vi "Collect_Info.vi"(5 "HART ports":refnum<visa-resource-name>[](array[refnum]), 7 "485 Ports":refnum<visa-resource-name>[](array[refnum]), 10 "MODBUS Serial Parameters":T7={"Mode"=enum."RTU", "Default Slave Address"=111, "MODBUS timeout"=1000, "Baud Rate"=38400, "Parity"=0, "Flow Control"=0} {"Flow Control" items=["None", "XON/XOFF", "RTS/CTS", "XON/XOFF & RTS/CTS", "DTR/DSR", "XON/XOFF & DTR/DSR"]; "Parity" items=["None", "Odd", "Even", "Mark", "Space"]}) -> (1 "Read Completed":bool, 2 "Information":T8, 3 "Byte order":T1(ring))   [LabVIEW 2016]
uses:
  Controls/Flow Tube Material.ctl
  Controls/mass flow unit codes.ctl
  Controls/Density Unit codes.ctl
  Controls/Temperature units.ctl
  Controls/Flow direction codes.ctl
  Controls/Information_tab_type.ctl
  OPC Server/MODBUS/MODBUS parameters type.ctl
  <vilib>/DeviceNet/VIAPI/subVIs/DnetIntfConfig.ctl
  OPC Server/Typedef/Array_of_Comm_mode_and_address_types.ctl
  OPC Server/Typedef/Comm_mode_and_address_type.ctl
  OPC Server/Typedef/Comm_mode_type_combo.ctl
  OPC Server/Protocol Class/Protocol.lvclass
  OPC Server/MASTER_OPC.ctl
  OPC Server/Typedef/event var.ctl
  OPC Server/Typedef/Comm ui action type.ctl
  OPC Server/Typedef/Comm_State_enum.ctl
  OPC Server/Typedef/state var.ctl
  OPC Server/MODBUS/MODBUS Class/MODBUS.lvclass
  C:/Users/d/Desktop/Software/Micromotion/Mark Lee/Source (1.10 US LV 2016) Branch Rabi/Blackbox/OPC Server/Protocol Class/Protocol.lvclass
  OPC Server/HART/HART Class/HART.lvclass
  OPC Server/Profibus/Profibus Class/Profibus.lvclass
  OPC Server/DeviceNET/DeviceNET Class/DeviceNET.lvclass
  OPC Server/Typedef/Protocol_enum_type.ctl
  <vilib>/DeviceNet/DeviceNetLIB.lvlib
panel:
  in  "MDOT":string="H2O"
  in  "Meter inlet static pressure (psia)":dbl
  in  "Fluid":string="H2O"
  in  "Product code*":string
  in  "Order number":string
  in  "Status *":enum32{"As found", "As left"}(radio)
  in  "Ref meter serial number*":string
  in  "Technician Name*":string
  in  "Customer Address":string
  in  "Customer Name":string
  in  "Done":bool
  out "status":bool
  in  "Protocol selection\n(appended)":T2=[{"address"=111, "Mode"=0}, {"address"=0, "Mode"=2}] {"Mode" items=["MODBUS", "HART", ""]}
  in  "Interface Name":T5(ring)
  in  "DeviceNet Interface Configuration":T6={"interface MAC ID"=0, "baud rate"=enum."500000", "poll mode"=enum."Automatic"} {"interface MAC ID" max=63 step=1}
  in  "Profibus Baud rate":i32(listbox)=6
  in  "Profibus ResourceName":refnum<visa-resource-name>="PXI5::11::INSTR"
  in  "Read":bool
  in  "Test Comments":string
  out "Test date and time":string
  out "Meter Zero":string
  in  "Meter Nominal Flow Rate (kg/min)*":string
  in  "Meter Density Repeatability":string
  in  "Meter Density Accuracy":string
  in  "Meter Zero Stability (kg/min) *":string
  in  "Meter flow repeatability":string
  in  "Meter flow accuracy (%) *":string
  out "Frequency span":string
  out "Frequency flow rate":string
  out "Flow direction":T9 items=["Forward flow only", "Reverse flow only", "Bidirectiona flow", "Absolute forward/reverse", "Negate/Forward only", "Negate/Bidirectional"]
  out "Mass flow damping":string
  out "Mass flow cutoff":string
  out "Temperature Units":T10 items=["Degrees Celsius"=32, "Degrees Fahrenheit"=33, "Degrees Rankine"=34, "Degrees Kelvin"=35, ""=0]
  out "Density units":T11 items=["Specific gravity units"=90, "Grams/cubic centimeter"=91, "Kg/cubic meter"=92, "Pounds/US gallon"=93, "Pounds/cubic foot"=94, "Grams/milliliter"=95, "Kg/liter"=96, "Pounds/cubic inch"=98, "Short tons/cubic yard"=99, "Degrees Baume (heavy)"=102, "Degrees Baume (light)"=103, "Degrees API"=104]
  out "Mass flow units":T12 items=["Grams/second"=70, "Grams/minute"=71, "Grams/hour"=72, "Kg/second"=73, "Kg/minute"=74, "Kg/hour"=75, "Kg/day"=76, "Metric tons/minute"=77, "Metric tons/hour"=78, "Metric tons/day"=79, "Pounds/second"=80, "Pounds/minute"=81, "Pounds/hour"=82, "Pounds/day"=83, "Short tons/minute"=84, "Short tons/hour"=85, "Short tons/day"=86, "Long tons/hour"=87, "Long tons/day"=88, "Special"=253]
  out "Transmitter Model":string
  in  "Sensor Model #":string
  in  "Transmitter Serial Number":string
  out "Density Temp Coeff":string
  out "FD":string
  out "K2":string
  out "K1":string
  out "D2":string
  out "D1":string
  out "FCF":string
  in  "Temp Rating":string
  in  "Pressure Rating":string
  out "Sensor Serial Number":string
  out "Flow Tube Material":T13 items=["Hastelloy C-22"=3, "Monel"=4, "Tantalum"=5, "Titanium"=6, "316L Stainless Steel"=19, "Inconel"=23, "Unknown"=252, "Special"=253]
  in  "Size":string
  # "Customer Information"
  # "*Required"
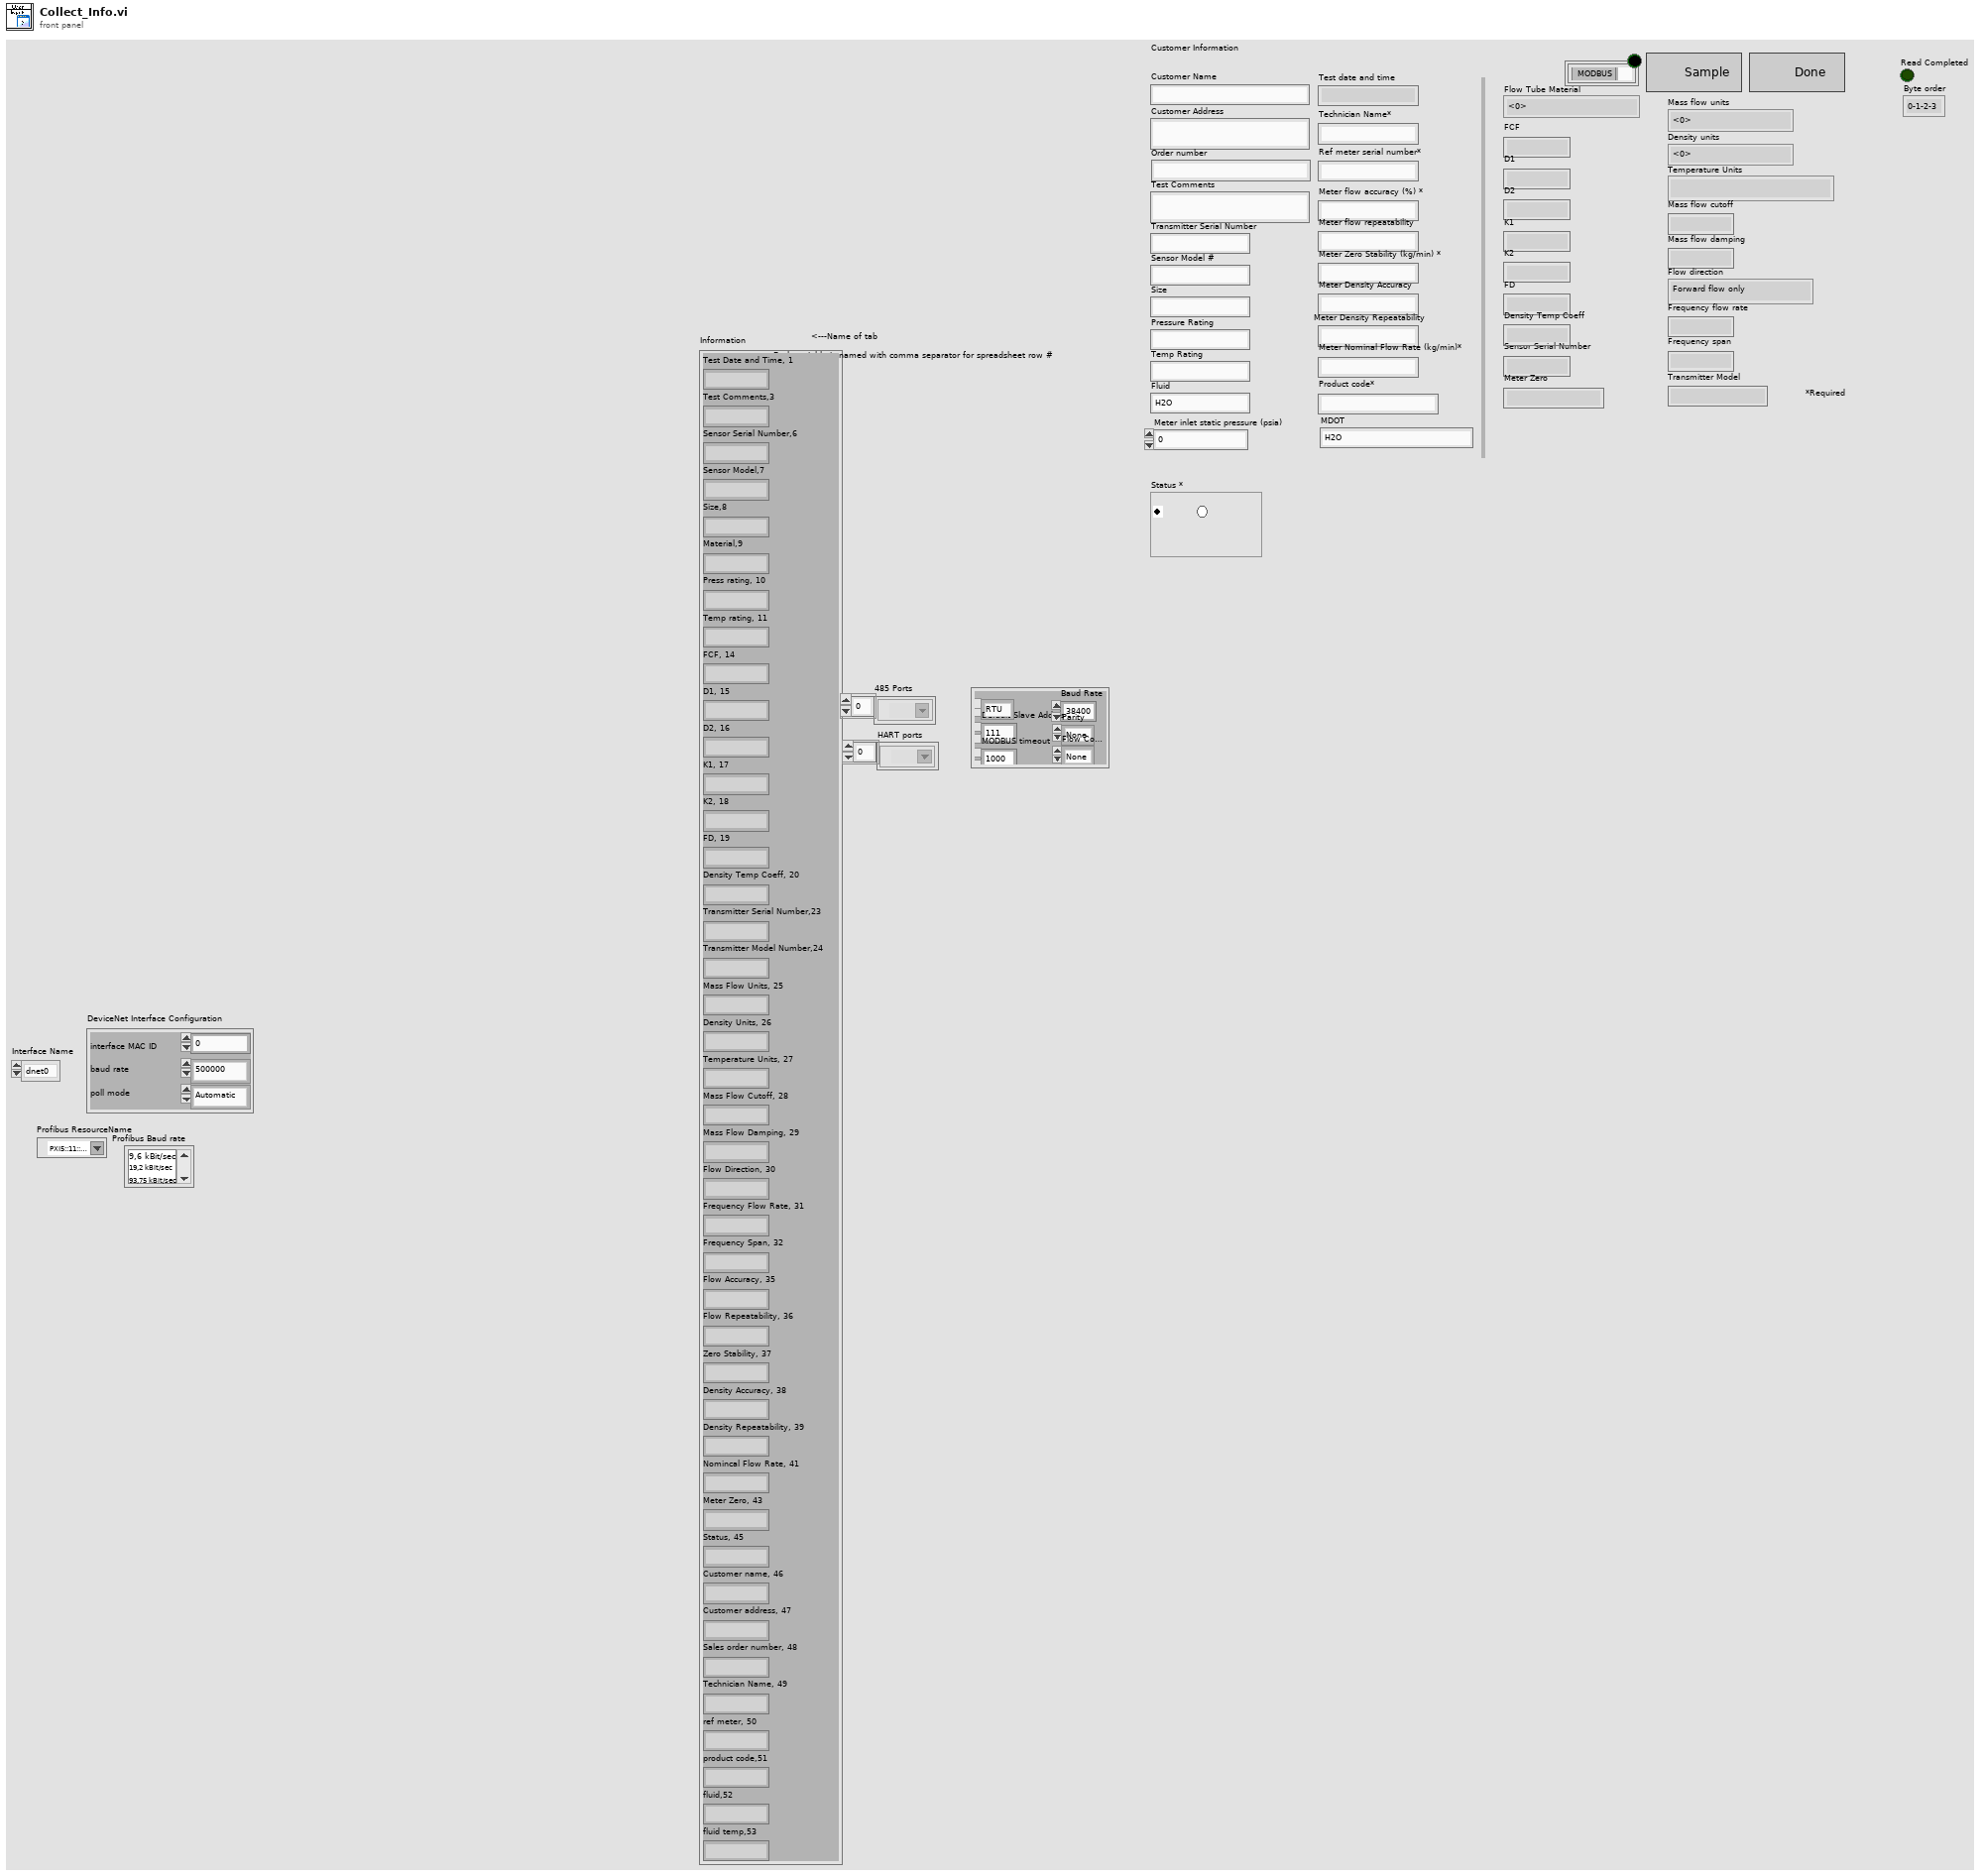
[diagram p1: front panel]
types:
  T1 = enum16{"0-1-2-3", "2-3-0-1", "1-0-3-2", "3-2-1-0"}
  T2 = typedef "Array_of_Comm_mode_and_address_types.ctl" = T3[]
  T3 = typedef "Comm_mode_and_address_type.ctl" = cluster{"address":i32, "Mode":T4}
  T4 = typedef "Comm_mode_type_combo.ctl" = u16
  T5 = enum16{"dnet0", "dnet1", "dnet2", "dnet3", "dnet4", "dnet5", "dnet6", "dnet7", "dnet8", "dnet9", "dnet10", "dnet11", "dnet12", "dnet13", "dnet14", "dnet15", "dnet16", "dnet17", "dnet18", "dnet19", "dnet20", "dnet21", "dnet22", "dnet23", "dnet24", "dnet25", "dnet26", "dnet27", "dnet28", "dnet29", "dnet30", "dnet31"}
  T6 = typedef "DeviceNetLIB.lvlib/DnetIntfConfig.ctl" = cluster{"interface MAC ID":u32, "baud rate":enum32{"125000", "250000", "500000"}, "poll mode":enum32{"Automatic", "Scanned", "Individual"}}
  T7 = typedef "MODBUS parameters type.ctl" = cluster{"Mode":enum16{"RTU", "ASCII"}, "Default Slave Address":u8, "MODBUS timeout":u32, "Baud Rate":u32, "Parity":u16, "Flow Control":u16}
  T8 = typedef "Information_tab_type.ctl" = cluster{"Test Date and Time, 1":string, "Test Comments,3":string, "Sensor Serial Number,6":string, "Sensor Model,7":string, "Size,8":string, "Material,9":string, "Press rating, 10":string, "Temp rating, 11":string, "FCF, 14":string, "D1, 15":string, "D2, 16":string, "K1, 17":string, "K2, 18":string, "FD, 19":string, "Density Temp Coeff, 20":string, "Transmitter Serial Number,23":string, "Transmitter Model Number,24":string, "Mass Flow Units, 25":string, "Density Units, 26":string, "Temperature Units, 27":string, "Mass Flow Cutoff, 28":string, "Mass Flow Damping, 29":string, "Flow Direction, 30":string, "Frequency Flow Rate, 31":string, "Frequency Span, 32":string, "Flow Accuracy, 35":string, "Flow Repeatability, 36":string, "Zero Stability, 37":string, "Density Accuracy, 38":string, "Density Repeatability, 39":string, "Nomincal Flow Rate, 41":string, "Meter Zero, 43":string, "Status, 45":string, "Customer name, 46":string, "Customer address, 47":string, "Sales order number, 48":string, "Technician Name, 49":string, "ref meter, 50":string, "product code,51":string, "fluid,52":string, "fluid temp,53":string}
  T9 = typedef "Flow direction codes.ctl" = u16
  T10 = typedef "Temperature units.ctl" = u16
  T11 = typedef "Density Unit codes.ctl" = u16
  T12 = typedef "mass flow unit codes.ctl" = u16
  T13 = typedef "Flow Tube Material.ctl" = u16
  T14 = typedef "MASTER_OPC.ctl" = cluster{"Main event var":refnum<user-event>, "VIRef":refnum<vi>, "Data path":path, "Reads":i32, "total number of UUT":i32, "FF refnum":cluster{"Handle1":u32, "Handle2":u32}, "FF device id list":string[], "MODBUS resource name":refnum<visa-resource-name>, "MODBUS Serial Parameters":cluster{"Mode":enum16{"RTU", "ASCII"}, "Default Slave Address":u8, "MODBUS timeout":u32, "Baud Rate":u32, "Parity":u16, "Flow Control":u16}, "Profibus resource name":refnum<visa-resource-name>, "Profibus Communication ref.:":u8, "HART resource name":refnum<visa-resource-name>, "HART long addresses (array)":u8[][], "Comm relay session":refnum<k15>, "Comm UI event":refnum<user-event>, "Write Interval (s)":dbl, "DMM_QUEUE":refnum<queue>, "POWER_QUEUE":refnum<queue>, "\nTHERM_QUEUE":refnum<queue>, "\nCOMM_QUEUE":refnum<queue>, "TIMING_QUEUE":refnum<queue>, "MAIN_QUEUE":refnum<queue>, "Log path":path}
  T15 = typedef "Protocol_enum_type.ctl" = enum16{"None", "MODBUS", "HART", "Fieldbus", "Profibus DP", "Profibus PA", "DeviceNET", "USB"}
  T16 = typedef "comm_variable_definition.ctl" = cluster{"General Parameter name":string, "MODBUS Register":i32, "Profibus":cluster{"Friendly name":string, "PA":cluster{"Slot":i32, "Index":i32}, "DP":cluster{"Slot":i32, "Index":i32}, "Tag":string}, "Fieldbus":cluster{"Parameter name":string, "Fieldbus Block":string, "Fieldbus Tag":string}, "data type":enum16{"float", "UINT", "UINT32", "STRING"}, "DeviceNET":cluster{"ClassId":u16, "InstanceId":u16, "AttributeId":u8}, "Cluster":T3, "Length":i32}
  T17 = cluster{"U16":u16, "U32":u32, "float":sgl, "string":string}
  T18 = typedef "CS_PB_DPV1_MSAC2_InitiateReqData.ctl" = cluster{"Communication ref.:":u8, "Send timeout:":u16, "Feat. supp. 1:":u8, "Feat. supp. 2:":u8, "Profile feat. supp. 1:":u8, "Profile feat. supp. 2:":u8, "Profile ID number:":u16, "Addional address parameter":cluster{"S-Type":bool, "S-Length:":u8, "D-Type":bool, "D-Length:":u8, "Data:":u8[]}}
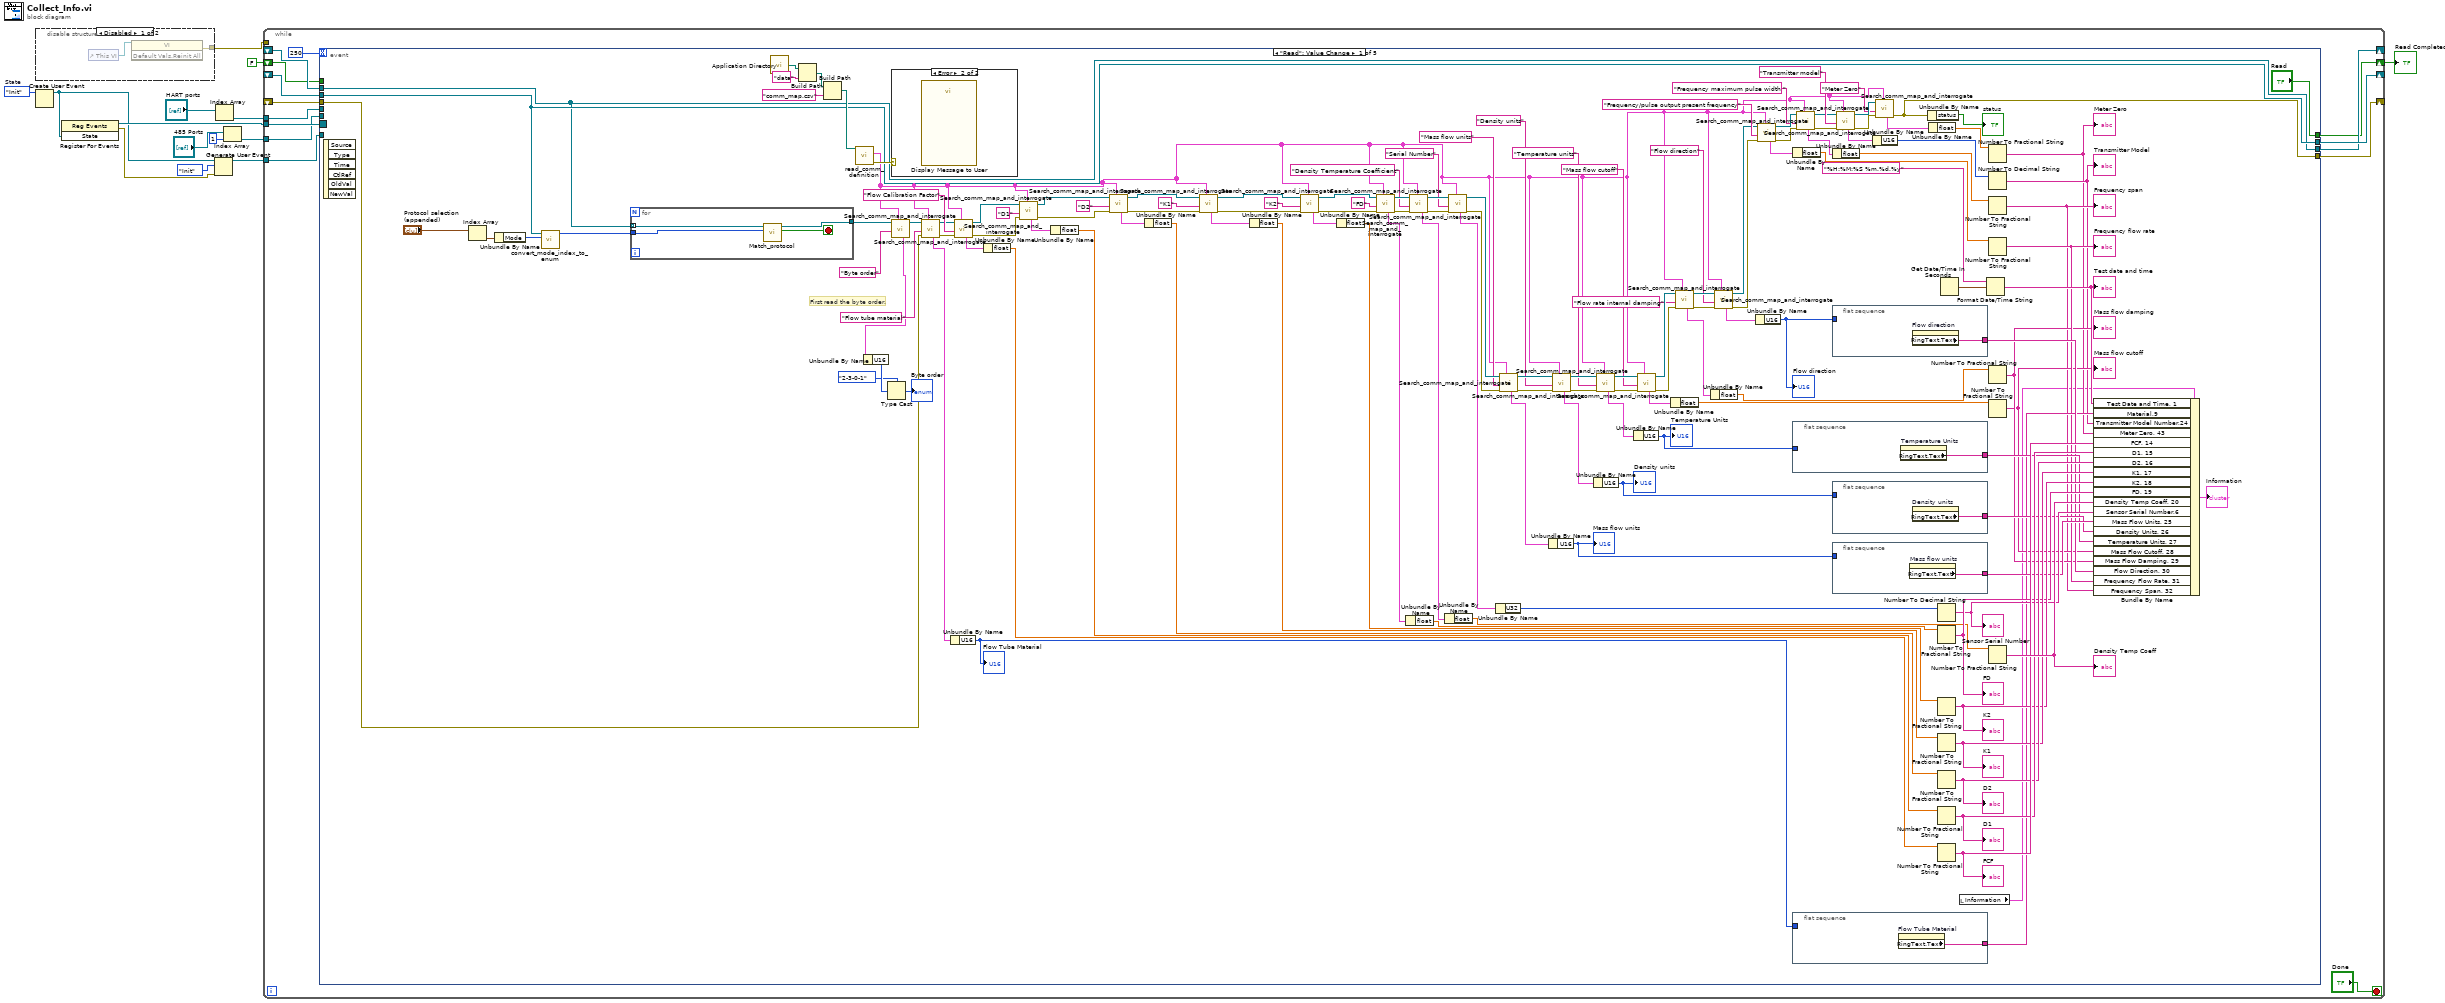
[diagram p0: block diagram]
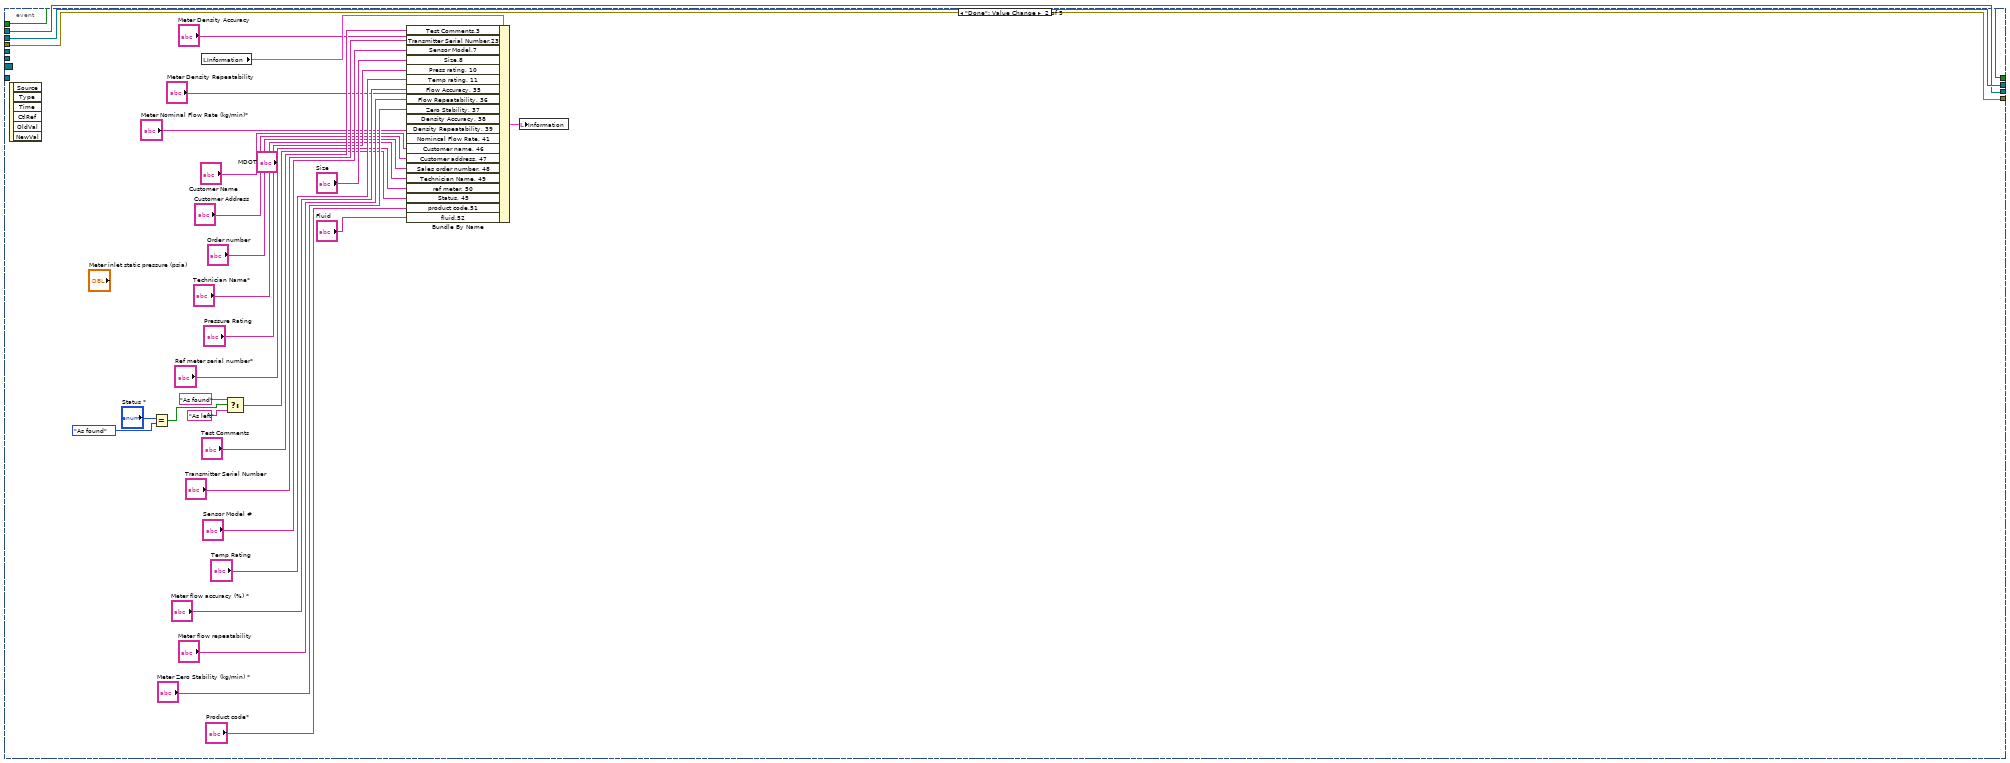
[diagram p4: hidden frame]
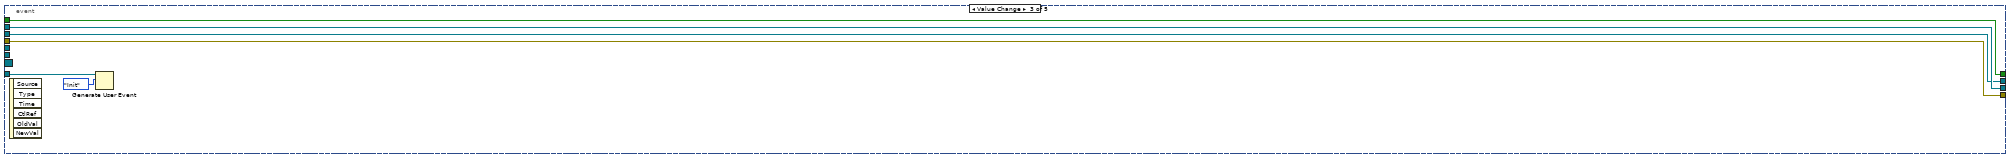
[diagram p5: hidden frame]
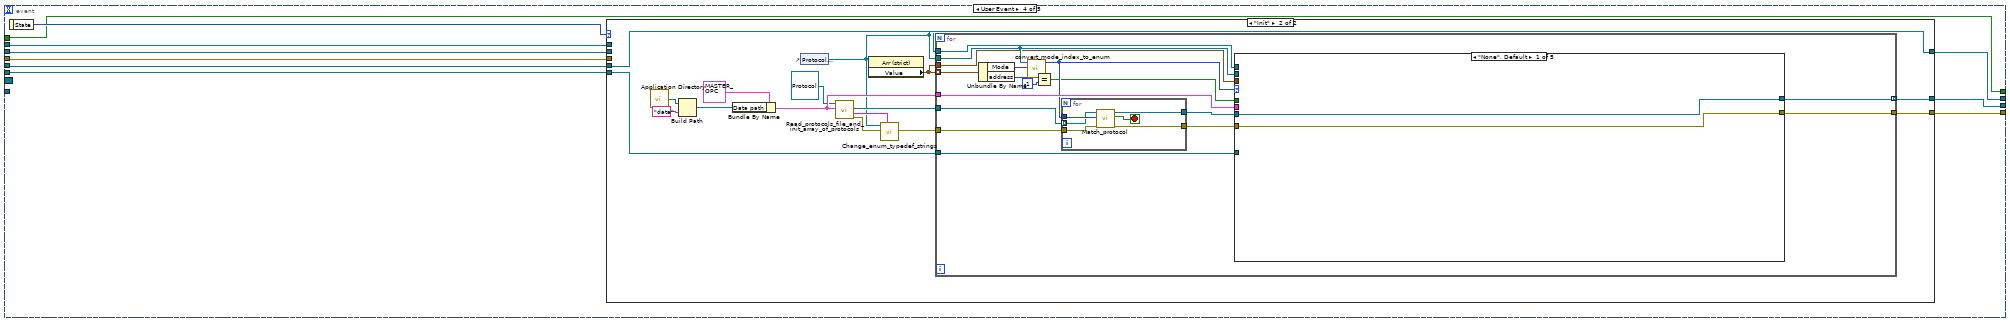
[diagram p6: hidden frame]
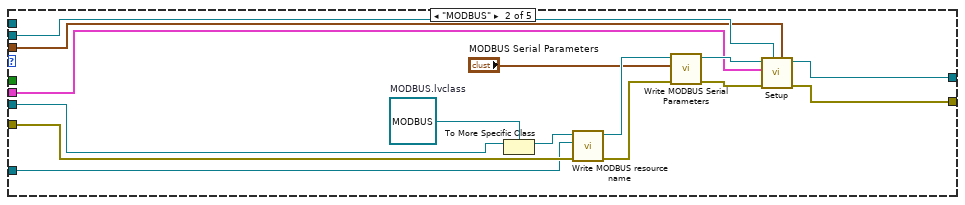
[diagram p8: hidden frame]
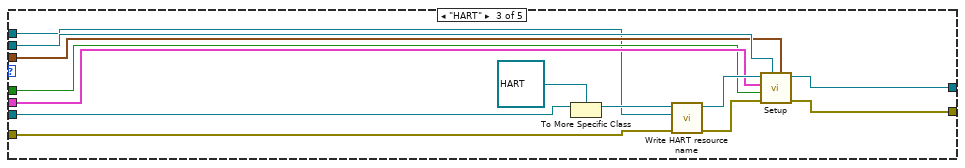
[diagram p9: hidden frame]
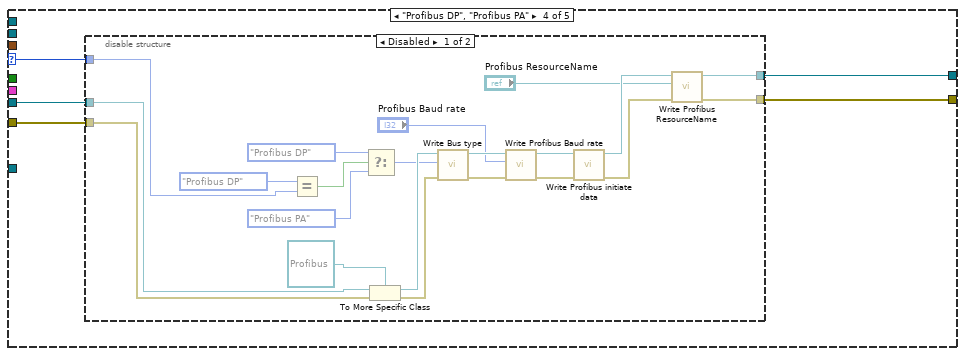
[diagram p10: hidden frame]
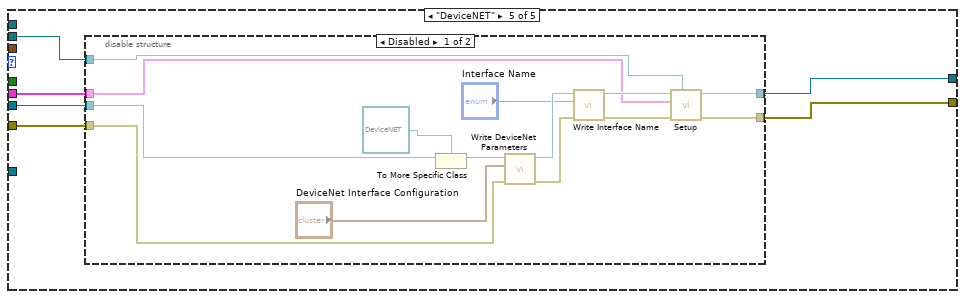
[diagram p12: hidden frame]
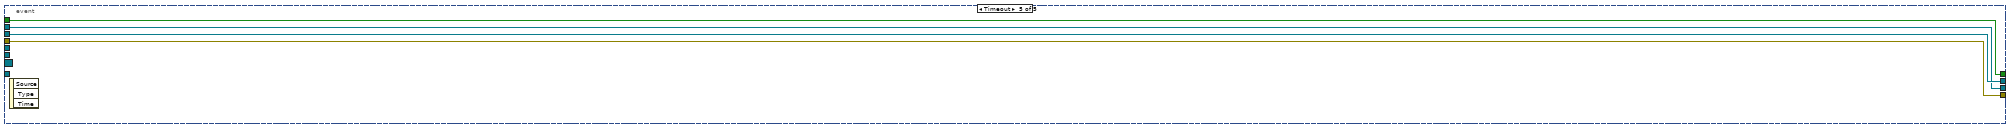
[diagram p14: hidden frame]
diagram:
  w9 = enum16{"Init", "Idle"}."Init"  # State
  n1 = disable-structure shown="Disabled" {
    disable-tunnel: [w15 _] -> w6
    frame Disabled {
      n2 = control-ref of="This VI"() -> (w16:refnum<vi>)
      n3 = invoke class="VI" method="Default Vals.Reinit All"(reference=w16) -> (error out=w15:errorcluster)  [unwired: 2 in, 2 out]
    }
    frame Enabled {
    }
  }
  n4 = Create User Event(user event datatype=w9) -> (user event=w10:refnum<user-event>)  [unwired: 1 in, 1 out]
  n5 = register-events(w10) -> (reference out=w12:refnum<event-registration>, error out=w14:errorcluster)  [unwired: 2 in]
  n6 = Generate User Event(user event=w10, event data cluster=enum16{"Init", "Idle"}."Init" ("event data"), error in=w14) -> (user event out=w11:refnum<user-event>)  [unwired: 1 in, 1 out]
  n7 = Index Array(array="HART ports") -> (element=w4:refnum<visa-resource-name>)  [unwired: 1 in]
  n8 = Index Array(array="485 Ports", index=1) -> (element=w2:refnum<visa-resource-name>)
  n9 = while {
    tunnel: w12 -> [w25]
    shift-right: [w24] -> _
    shift-left: _ -> [w28]
    shift-right: [w23] -> _
    shift-left: _ -> [w30]
    shift-right: [w22] -> _
    shift-left: _ -> [w29]
    tunnel: w11 -> [w21]
    shift-right: [w20] -> w8
    shift-left: FALSE ("Read") -> [w19]
    tunnel: w6 -> [_]
    tunnel: w4 -> [w18]
    tunnel: w2 -> [w17]
    stop <- "Done" stop-if-true
    n10 = event shown="[0] \"Read\": Value Change" {
      selector: w25 -> [_ _ _ _ _]
      dyn-events: _ -> [_ _ _ _ _]
      timeout: u32 250 ("millisecond multiple") -> [_ _ _ _ _]
      tunnel: w30 -> [w40 w210 w215 w223 w349]
      tunnel: w29 -> [w171 w209 w213 w222 w348]
      tunnel: w28 -> [w42 w211 w214 w221 w350]
      tunnel: [w42 w211 w214 w227 w350] -> w24
      tunnel: [w40 w210 w215 w226 w349] -> w23
      tunnel: [w169 w209 w213 w225 w348] -> w22
      tunnel: w21 -> [_ _ w217 _ _]
      tunnel: ["Read" w208 w212 w220 w347] -> w20
      tunnel: w19 -> [_ w208 w212 w220 w347]
      tunnel: w18 -> [_ _ _ w219 _]
      tunnel: w17 -> [_ _ _ w218 _]
      event "Read": Value Change {
        # "First read the byte order."
        n11 = event-data() -> ()  [unwired: 1 in, 6 out]
        n12 = Index Array(array="Protocol selection\n(appended)") -> (element=w44:T3)  [unwired: 1 in]
        n13 = Unbundle By Name(w44) -> ("Mode"=w43:T4)
        n14 = call "convert_mode_index_to_enum.vi"("index"=w43, "CtlRef"=w42) -> ("Protocol enum"=w41:T15)  [unwired: 6 in, 3 out]
        n15 = for {
          tunnel: w41 -> [w175]
          tunnel: w40 -> [w174] mode=indexing
          tunnel: [w172] -> w38
          stop <- w173 stop-if-true
          n16 = call-dynamic "Match_protocol.vi"("Protocol type"=w175, "Protocol in"=w174) -> ("Match"=w173:bool, "Protocol out"=w172:refnum<class "Protocol.lvclass">)  [unwired: 7 in, 1 out]
        }
        n17 = call <vilib>:"Application Directory.vi"() -> ("Application Directory"=w163:path)
        n18 = Build Path(base path=w163, name or relative path="data") -> (appended path=w159:path)
        n19 = Build Path(base path=w159, name or relative path="comm_map.csv") -> (appended path=w161:path)
        n20 = call "read_comm_definition.vi"("file path (dialog if empty)"=w161) -> ("error out"=w158:errorcluster, "Comm variable definitions"=w36:T16[])  [unwired: 8 in, 1 out]
        n21 = case shown="Error" w158 {
          frame No Error {
          }
          frame Error {
            n22 = call "Display Message to User"() -> ()  [unwired: 10 in, 2 out]
          }
        }
        n23 = call "Search_comm_map_and_interrogate.vi"("array of registers"=w36, "Register name"="Byte order", "Protocol in"=w38) -> ("Protocol out"=w37:refnum<class "Protocol.lvclass">, "output cluster"=w34:T17)  [unwired: 6 in, 1 out]
        n24 = Unbundle By Name(w34) -> ("U16"=w33:u16)
        n25 = Type Cast(type=T1."2-3-0-1" ("Byte order"), x=w33) -> (*(type *) &x=→"Byte order":T1)
        n26 = call "Search_comm_map_and_interrogate.vi"("array of registers"=w36, "error in (no error)"=w171, "Register name"="Flow tube material", "Protocol in"=w37) -> ("error out"=w78:errorcluster, "Protocol out"=w79:refnum<class "Protocol.lvclass">, "output cluster"=w77:T17)  [unwired: 5 in]
        n27 = Unbundle By Name(w77) -> ("U16"=w74:u16)
        "Flow Tube Material" <- w74
        n28 = call "Search_comm_map_and_interrogate.vi"("array of registers"=w36, "error in (no error)"=w78, "Register name"="Flow Calibration Factor", "Protocol in"=w79) -> ("error out"=w156:errorcluster, "Protocol out"=w155:refnum<class "Protocol.lvclass">, "output cluster"=w153:T17)  [unwired: 5 in]
        n29 = Unbundle By Name(w153) -> ("float"=w152:sgl)
        n30 = call "Search_comm_map_and_interrogate.vi"("array of registers"=w36, "error in (no error)"=w156, "Register name"="D1", "Protocol in"=w155) -> ("error out"=w150:errorcluster, "Protocol out"=w154:refnum<class "Protocol.lvclass">, "output cluster"=w147:T17)  [unwired: 5 in]
        n31 = Unbundle By Name(w147) -> ("float"=w148:sgl)
        n32 = call "Search_comm_map_and_interrogate.vi"("array of registers"=w36, "error in (no error)"=w150, "Register name"="D2", "Protocol in"=w154) -> ("error out"=w140:errorcluster, "Protocol out"=w141:refnum<class "Protocol.lvclass">, "output cluster"=w143:T17)  [unwired: 5 in]
        n33 = Unbundle By Name(w143) -> ("float"=w144:sgl)
        n34 = call "Search_comm_map_and_interrogate.vi"("array of registers"=w36, "error in (no error)"=w140, "Register name"="K1", "Protocol in"=w141) -> ("error out"=w134:errorcluster, "Protocol out"=w135:refnum<class "Protocol.lvclass">, "output cluster"=w138:T17)  [unwired: 5 in]
        n35 = Unbundle By Name(w138) -> ("float"=w139:sgl)
        n36 = call "Search_comm_map_and_interrogate.vi"("array of registers"=w36, "error in (no error)"=w134, "Register name"="K2", "Protocol in"=w135) -> ("error out"=w128:errorcluster, "Protocol out"=w129:refnum<class "Protocol.lvclass">, "output cluster"=w131:T17)  [unwired: 5 in]
        n37 = Unbundle By Name(w131) -> ("float"=w132:sgl)
        n38 = call "Search_comm_map_and_interrogate.vi"("array of registers"=w36, "error in (no error)"=w128, "Register name"="FD", "Protocol in"=w129) -> ("error out"=w121:errorcluster, "Protocol out"=w123:refnum<class "Protocol.lvclass">, "output cluster"=w127:T17)  [unwired: 5 in]
        n39 = Unbundle By Name(w127) -> ("float"=w125:sgl)
        n40 = call "Search_comm_map_and_interrogate.vi"("array of registers"=w36, "error in (no error)"=w121, "Register name"="Density Temperature Coefficient", "Protocol in"=w123) -> ("error out"=w118:errorcluster, "Protocol out"=w117:refnum<class "Protocol.lvclass">, "output cluster"=w119:T17)  [unwired: 5 in]
        n41 = Unbundle By Name(w119) -> ("float"=w120:sgl)
        n42 = call "Search_comm_map_and_interrogate.vi"("array of registers"=w36, "error in (no error)"=w118, "Register name"="Serial Number", "Protocol in"=w117) -> ("error out"=w112:errorcluster, "Protocol out"=w113:refnum<class "Protocol.lvclass">, "output cluster"=w115:T17)  [unwired: 5 in]
        n43 = Unbundle By Name(w115) -> ("U32"=w59:u32)
        n44 = call "Search_comm_map_and_interrogate.vi"("array of registers"=w36, "error in (no error)"=w112, "Register name"="Mass flow units", "Protocol in"=w113) -> ("error out"=w111:errorcluster, "Protocol out"=w110:refnum<class "Protocol.lvclass">, "output cluster"=w108:T17)  [unwired: 5 in]
        n45 = Unbundle By Name(w108) -> ("U16"=w104:u16)
        "Mass flow units" <- w104
        n46 = call "Search_comm_map_and_interrogate.vi"("array of registers"=w36, "error in (no error)"=w111, "Register name"="Density units", "Protocol in"=w110) -> ("error out"=w100:errorcluster, "Protocol out"=w101:refnum<class "Protocol.lvclass">, "output cluster"=w106:T17)  [unwired: 5 in]
        n47 = Unbundle By Name(w106) -> ("U16"=w102:u16)
        "Density units" <- w102
        n48 = call "Search_comm_map_and_interrogate.vi"("array of registers"=w36, "error in (no error)"=w100, "Register name"="Temperature units", "Protocol in"=w101) -> ("error out"=w95:errorcluster, "Protocol out"=w94:refnum<class "Protocol.lvclass">, "output cluster"=w98:T17)  [unwired: 5 in]
        n49 = Unbundle By Name(w98) -> ("U16"=w97:u16)
        "Temperature Units" <- w97
        n50 = call "Search_comm_map_and_interrogate.vi"("array of registers"=w36, "error in (no error)"=w95, "Register name"="Mass flow cutoff", "Protocol in"=w94) -> ("error out"=w88:errorcluster, "Protocol out"=w90:refnum<class "Protocol.lvclass">, "output cluster"=w92:T17)  [unwired: 5 in]
        n51 = Unbundle By Name(w92) -> ("float"=w91:sgl)
        n52 = call "Search_comm_map_and_interrogate.vi"("array of registers"=w36, "error in (no error)"=w88, "Register name"="Flow rate internal damping", "Protocol in"=w90) -> ("error out"=w84:errorcluster, "Protocol out"=w85:refnum<class "Protocol.lvclass">, "output cluster"=w87:T17)  [unwired: 5 in]
        n53 = Unbundle By Name(w87) -> ("float"=w86:sgl)
        n54 = call "Search_comm_map_and_interrogate.vi"("array of registers"=w36, "error in (no error)"=w84, "Register name"="Flow direction", "Protocol in"=w85) -> ("error out"=w73:errorcluster, "Protocol out"=w58:refnum<class "Protocol.lvclass">, "output cluster"=w82:T17)  [unwired: 5 in]
        n55 = Unbundle By Name(w82) -> ("U16"=w81:u16)
        "Flow direction" <- w81
        n56 = call "Search_comm_map_and_interrogate.vi"("array of registers"=w36, "error in (no error)"=w73, "Register name"="Frequency/pulse output present frequency", "Protocol in"=w58) -> ("error out"=w66:errorcluster, "Protocol out"=w67:refnum<class "Protocol.lvclass">, "output cluster"=w71:T17)  [unwired: 5 in]
        n57 = Unbundle By Name(w71) -> ("float"=w70:sgl)
        n58 = flat-sequence {
          tunnel: [w178] -> w96
          tunnel: w97 -> [_]
          frame #0 {
            n59 = property on="Temperature Units" class="Ring (strict)"() -> ("RingText.Text"=w178:string)  [unwired: 2 in, 2 out]
          }
        }
        n60 = flat-sequence {
          tunnel: [w176] -> w75
          tunnel: w74 -> [_]
          frame #0 {
            n61 = property on="Flow Tube Material" class="Ring (strict)"() -> ("RingText.Text"=w176:string)  [unwired: 2 in, 2 out]
          }
        }
        n62 = call "Search_comm_map_and_interrogate.vi"("array of registers"=w36, "error in (no error)"=w66, "Register name"="Frequency maximum pulse width ", "Protocol in"=w67) -> ("error out"=w55:errorcluster, "Protocol out"=w56:refnum<class "Protocol.lvclass">, "output cluster"=w64:T17)  [unwired: 5 in]
        n63 = Unbundle By Name(w64) -> ("float"=w63:sgl)
        n64 = flat-sequence {
          tunnel: w81 -> [_]
          tunnel: [w177] -> w80
          frame #0 {
            n65 = property on="Flow direction" class="Ring (strict)"() -> ("RingText.Text"=w177:string)  [unwired: 2 in, 2 out]
          }
        }
        n66 = flat-sequence {
          tunnel: [w179] -> w103
          tunnel: w102 -> [_]
          frame #0 {
            n67 = property on="Density units" class="Ring (strict)"() -> ("RingText.Text"=w179:string)  [unwired: 2 in, 2 out]
          }
        }
        n68 = flat-sequence {
          tunnel: [w180] -> w105
          tunnel: w104 -> [_]
          frame #0 {
            n69 = property on="Mass flow units" class="Ring (strict)"() -> ("RingText.Text"=w180:string)  [unwired: 2 in, 2 out]
          }
        }
        n70 = call "Search_comm_map_and_interrogate.vi"("array of registers"=w36, "error in (no error)"=w55, "Register name"="Transmitter model", "Protocol in"=w56) -> ("error out"=w51:errorcluster, "Protocol out"=w50:refnum<class "Protocol.lvclass">, "output cluster"=w54:T17)  [unwired: 5 in]
        n71 = Unbundle By Name(w54) -> ("U16"=w53:u16)
        n72 = call "Search_comm_map_and_interrogate.vi"("array of registers"=w36, "error in (no error)"=w51, "Register name"="Meter Zero", "Protocol in"=w50) -> ("error out"=w169:errorcluster, "output cluster"=w48:T17)  [unwired: 5 in, 1 out]
        n73 = Unbundle By Name(w169) -> ("status"=→"status":bool)
        n74 = Unbundle By Name(w48) -> ("float"=w47:sgl)
        n75 = Number To Decimal String(number=w59) -> (decimal integer string=w114:string)  [unwired: 1 in]
        "Sensor Serial Number" <- w114
        n76 = Number To Fractional String(number=w125) -> (F-format string=w124:string)  [unwired: 3 in]
        "FD" <- w124
        n77 = Number To Fractional String(number=w132) -> (F-format string=w130:string)  [unwired: 3 in]
        "K2" <- w130
        n78 = Number To Fractional String(number=w139) -> (F-format string=w136:string)  [unwired: 3 in]
        "K1" <- w136
        n79 = Number To Fractional String(number=w144) -> (F-format string=w142:string)  [unwired: 3 in]
        "D2" <- w142
        n80 = Number To Fractional String(number=w148) -> (F-format string=w146:string)  [unwired: 3 in]
        "D1" <- w146
        n81 = Number To Fractional String(number=w152) -> (F-format string=w151:string)  [unwired: 3 in]
        "FCF" <- w151
        n82 = Get Date/Time In Seconds() -> (seconds since 1Jan1904=w168:timestamp)
        n83 = local read "Information"() -> (w39:T8)
        n84 = Format Date/Time String(time format string (%c)="%H:%M:%S %m.%d.%y", seconds (now)=w168) -> (date/time string=w166:string)  [unwired: 1 in]
        "Test date and time" <- w166
        n85 = Number To Fractional String(number=w47) -> (F-format string=w46:string)  [unwired: 3 in]
        "Meter Zero" <- w46
        n86 = Number To Decimal String(number=w53) -> (decimal integer string=w52:string)  [unwired: 1 in]
        "Transmitter Model" <- w52
        n87 = Number To Fractional String(number=w63) -> (F-format string=w61:string)  [unwired: 3 in]
        "Frequency span" <- w61
        n88 = Number To Fractional String(number=w70) -> (F-format string=w69:string)  [unwired: 3 in]
        "Frequency flow rate" <- w69
        n89 = Number To Fractional String(number=w86) -> (F-format string=w68:string)  [unwired: 3 in]
        "Mass flow damping" <- w68
        n90 = Number To Fractional String(number=w91) -> (F-format string=w62:string)  [unwired: 3 in]
        "Mass flow cutoff" <- w62
        n91 = Number To Fractional String(number=w120) -> (F-format string=w165:string)  [unwired: 3 in]
        "Density Temp Coeff" <- w165
        n92 = Bundle By Name(cluster=w39, "Test Date and Time, 1"=w166, "Material,9"=w75, "Transmitter Model Number,24"=w52, "Meter Zero, 43"=w46, "FCF, 14"=w151, "D1, 15"=w146, "D2, 16"=w142, "K1, 17"=w136, "K2, 18"=w130, "FD, 19"=w124, "Density Temp Coeff, 20"=w165, "Sensor Serial Number,6"=w114, "Mass Flow Units, 25"=w105, "Density Units, 26"=w103, "Temperature Units, 27"=w96, "Mass Flow Cutoff, 28"=w62, "Mass Flow Damping, 29"=w68, "Flow Direction, 30"=w80, "Frequency Flow Rate, 31"=w69, "Frequency Span, 32"=w61) -> (→"Information":T8)
      }
      event "Done": Value Change {
        n93 = event-data() -> ()  [unwired: 1 in, 6 out]
        n94 = Equal?(x="Status *", y=enum32{"As found", "As left"}."As found") -> (x = y?=w193:bool)
        n95 = local read "Information"() -> (w207:T8)
        n96 = Select(t="As found" ("Technician Name*"), s=w193, f="As left") -> (s? t:f=w183:string)
        n97 = Bundle By Name(cluster=w207, "Test Comments,3"="Test Comments", "Transmitter Serial Number,23"="Transmitter Serial Number", "Sensor Model,7"="Sensor Model #", "Size,8"="Size", "Press rating, 10"="Pressure Rating", "Temp rating, 11"="Temp Rating", "Flow Accuracy, 35"="Meter flow accuracy (%) *", "Flow Repeatability, 36"="Meter flow repeatability", "Zero Stability, 37"="Meter Zero Stability (kg/min) *", "Density Accuracy, 38"="Meter Density Accuracy", "Density Repeatability, 39"="Meter Density Repeatability", "Nomincal Flow Rate, 41"="Meter Nominal Flow Rate (kg/min)*", "Customer name, 46"="Customer Name", "Customer address, 47"="Customer Address", "Sales order number, 48"="Order number", "Technician Name, 49"="Technician Name*", "ref meter, 50"="Ref meter serial number*", "Status, 45"=w183, "product code,51"="Product code*", "fluid,52"="Fluid") -> (w194:T8)
        n98 = local write "Information"(w194) -> ()
      }
      event Value Change {
        n99 = event-data() -> ()  [unwired: 1 in, 6 out]
        n100 = Generate User Event(user event=w217, event data cluster=enum16{"Init", "Idle"}."Init" ("event data")) -> ()  [unwired: 2 in, 2 out]
      }
      event User Event {
        n101 = event-data() -> ("State"=w224:enum16{"Init", "Idle"})  [unwired: 1 in]
        n102 = case shown="\"Init\"" w224 {
          tunnel: [w228 w234] -> w227
          tunnel: [w230 w236] -> w226
          tunnel: [w229 w235] -> w225
          tunnel: w223 -> [w230 _]
          tunnel: w222 -> [w229 _]
          tunnel: w221 -> [w228 _]
          tunnel: w219 -> [_ w232]
          tunnel: w218 -> [_ w231]
          frame "Idle", Default {
          }
          frame "Init" {
            n103 = call <vilib>:"Application Directory.vi"() -> ("Application Directory"=w243:path)
            n104 = Build Path(base path=w243, name or relative path="data") -> (appended path=w245:path)
            n105 = Bundle By Name(cluster=T14 {"Main event var"=refnum, "VIRef"=refnum, "Data path"=path "", "Reads"=0, "total number of UUT"=0, "FF refnum"={"Handle1"=0, "Handle2"=0}, "FF device id list"=[], "MODBUS resource name"="", "MODBUS Serial Parameters"={"Mode"=enum."RTU", "Default Slave Address"=0, "MODBUS timeout"=0, "Baud Rate"=0, "Parity"=0, "Flow Control"=0}, "Profibus resource name"="", "Profibus Communication ref.:"=0, "HART resource name"="", "HART long addresses (array)"=[], "Comm relay session"="", "Comm UI event"=refnum, "Write Interval (s)"=5.0, "DMM_QUEUE"=refnum, "POWER_QUEUE"=refnum, "\nTHERM_QUEUE"=refnum, "\nCOMM_QUEUE"=refnum, "TIMING_QUEUE"=refnum, "MAIN_QUEUE"=refnum, "Log path"=path ""} ("Comm master cluster"), "Data path"=w245) -> (w246:T14)
            n106 = control-ref of="Protocol selection\n(appended)"() -> (w234:refnum<vi>)
            n107 = call-dynamic "Read_protocols_file_and_init_array_of_protocols.vi"("Comm master cluster"=w246, "Protocol in"=refnum<class "Protocol.lvclass"> refnum) -> ("error out"=w240:errorcluster, "Array of configured protocols"=w239:string[], "Array of Protocols out"=w238:refnum<class "Protocol.lvclass">[])  [unwired: 6 in, 1 out]
            n108 = property class="Arr (strict)"(reference=w234) -> ("Value"=w233:T2)  [unwired: 1 in, 2 out]
            n109 = call "Change_enum_typedef_strings.vi"("Strings []"=w239, "error in (no error)"=w240, "protocol selection ref"=w234) -> ("error out"=w241:errorcluster)  [unwired: 8 in]
            n110 = for {
              tunnel: w238 -> [w257]
              tunnel: [w263] -> w236 mode=indexing
              tunnel: [w262] -> w235
              tunnel: w234 -> [w260]
              tunnel: w241 -> [w254]
              tunnel: w246 -> [w261]
              tunnel: w233 -> [w259] mode=indexing
              tunnel: w233 -> [w249]
              tunnel: w232 -> [w248]
              tunnel: w231 -> [w247]
              n111 = Unbundle By Name(w259) -> ("Mode"=w258:T4, "address"=w252:i32)
              n112 = call "convert_mode_index_to_enum.vi"("index"=w258, "CtlRef"=w260) -> ("Protocol enum"=w253:T15)  [unwired: 6 in, 3 out]
              n113 = Equal?(x=w252, y=-1) -> (x = y?=w250:bool)
              n114 = for {
                tunnel: [w269] -> w256
                tunnel: [w267] -> w255
                tunnel: w253 -> [w266]
                tunnel: w257 -> [w265] mode=indexing
                tunnel: w254 -> [w264]
                stop <- w268 stop-if-true
                n115 = call-dynamic "Match_protocol.vi"("error in (no error)"=w264, "Protocol type"=w266, "Protocol in"=w265) -> ("error out"=w267:errorcluster, "Match"=w268:bool, "Protocol out"=w269:refnum<class "Protocol.lvclass">)  [unwired: 6 in]
              }
              n116 = case shown="\"None\", Default" w253 {
                selector: w253 -> [_ _ _ w301 _]
                tunnel: w256 -> [w271 w286 w299 w304 w332]
                tunnel: [w271 w284 w295 w300 w331] -> w263
                tunnel: [w270 w277 w292 w303 w330] -> w262
                tunnel: w255 -> [w270 w276 w297 w302 w329]
                tunnel: w261 -> [_ w275 w294 _ w328]
                tunnel: w260 -> [_ w274 w291 _ w327]
                tunnel: w250 -> [_ _ w289 _ _]
                tunnel: w249 -> [_ w273 w288 _ _]
                tunnel: w248 -> [_ _ w287 _ _]
                tunnel: w247 -> [_ w272 _ _ _]
                frame "None", Default {
                }
                frame "MODBUS" {
                  w285 = refnum<class "MODBUS.lvclass"> refnum  # MODBUS.lvclass
                  n117 = To More Specific Class(target class=w285, reference=w286) -> (specific class reference=w283:refnum<class "MODBUS.lvclass">)  [unwired: 1 in, 1 out]
                  n118 = call-dynamic "Write MODBUS resource name.vi"("error in (no error)"=w276, "MODBUS resource name"=w272, "MODBUS in"=w283) -> ("error out"=w282:errorcluster, "MODBUS out"=w281:refnum<class "MODBUS.lvclass">)  [unwired: 7 in]
                  n119 = call-dynamic "Write MODBUS Serial Parameters.vi"("error in (no error)"=w282, "MODBUS Serial Parameters"="MODBUS Serial Parameters", "MODBUS in"=w281) -> ("error out"=w278:errorcluster, "MODBUS out"=w279:refnum<class "MODBUS.lvclass">)  [unwired: 7 in]
                  n120 = call-dynamic "Setup.vi"("Protocol selection\n(appended)"=w273, "protocol selection ref"=w274, "error in (no error)"=w278, "Comm master cluster in"=w275, "MODBUS in"=w279) -> ("error out"=w277:errorcluster, "MODBUS out"=w284:refnum<class "MODBUS.lvclass">)  [unwired: 5 in]
                }
                frame "HART" {
                  n121 = To More Specific Class(target class=refnum<class "HART.lvclass"> refnum ("HART.lvclass"), reference=w299) -> (specific class reference=w298:refnum<class "HART.lvclass">)  [unwired: 1 in, 1 out]
                  n122 = call-dynamic "Write HART resource name.vi"("error in (no error)"=w297, "HART resource name"=w287, "HART in"=w298) -> ("error out"=w293:errorcluster, "HART out"=w296:refnum<class "HART.lvclass">)  [unwired: 7 in]
                  n123 = call-dynamic "Setup.vi"("Protocol selection\n(appended)"=w288, "protocol selection ref"=w291, "error in (no error)"=w293, "search"=w289, "Comm master cluster in"=w294, "HART in"=w296) -> ("error out"=w292:errorcluster, "HART out"=w295:refnum<class "HART.lvclass">)  [unwired: 4 in]
                }
                frame "Profibus DP", "Profibus PA" {
                  n124 = disable-structure shown="Disabled" {
                    disable-tunnel: w304 -> [w325 _]
                    disable-tunnel: [w321 _] -> w303
                    disable-tunnel: w302 -> [w315 _]
                    disable-tunnel: w301 -> [w313 _]
                    disable-tunnel: [w305 _] -> w300
                    frame Disabled {
                      n125 = Equal?(x=Protocol_enum_type."Profibus DP" ("Protocols"), y=w313) -> (x = y?=w312:bool)
                      n126 = Select(t=enum16{"Profibus DP", "Profibus PA"}."Profibus DP" ("Bus type"), s=w312, f=enum16{"Profibus DP", "Profibus PA"}."Profibus PA" ("Bus type")) -> (s? t:f=w309:enum16{"Profibus DP", "Profibus PA"})
                      n127 = To More Specific Class(target class=refnum<class "Profibus.lvclass"> refnum ("Profibus.lvclass"), reference=w325, error in=w315) -> (specific class reference=w317:refnum<class "Profibus.lvclass">, error out=w316:errorcluster)
                      n128 = call-dynamic "Write Bus type.vi"("error in (no error)"=w316, "Bus type"=w309, "Profibus in"=w317) -> ("error out"=w324:errorcluster, "Profibus out"=w320:refnum<class "Profibus.lvclass">)  [unwired: 7 in]
                      n129 = call-dynamic "Write Profibus Baud rate.vi"("error in (no error)"=w324, "Profibus Baud rate"="Profibus Baud rate", "Profibus in"=w320) -> ("error out"=w323:errorcluster, "Profibus out"=w319:refnum<class "Profibus.lvclass">)  [unwired: 7 in]
                      n130 = call-dynamic "Write Profibus initiate data.vi"("error in (no error)"=w323, "Profibus in"=w319) -> ("error out"=w322:errorcluster, "Profibus out"=w318:refnum<class "Profibus.lvclass">, "Initiate data"=w307:T18)  [unwired: 7 in]
                      n131 = call-dynamic "Write Profibus ResourceName.vi"("error in (no error)"=w322, "Profibus ResourceName"="Profibus ResourceName", "Profibus in"=w318) -> ("error out"=w321:errorcluster, "Profibus out"=w305:refnum<class "Profibus.lvclass">)  [unwired: 7 in]
                    }
                    frame Enabled {
                    }
                  }
                }
                frame "DeviceNET" {
                  n132 = disable-structure shown="Disabled" {
                    disable-tunnel: w332 -> [w346 _]
                    disable-tunnel: [w345 _] -> w331
                    disable-tunnel: [w344 _] -> w330
                    disable-tunnel: w329 -> [w338 _]
                    disable-tunnel: w328 -> [w334 _]
                    disable-tunnel: w327 -> [w333 _]
                    frame Disabled {
                      n133 = To More Specific Class(target class=refnum<class "DeviceNET.lvclass"> refnum ("DeviceNET.lvclass"), reference=w346) -> (specific class reference=w335:refnum<class "DeviceNET.lvclass">)  [unwired: 1 in, 1 out]
                      n134 = call-dynamic "Write DeviceNet Parameters.vi"("error in (no error)"=w338, "DeviceNet Interface Configuration"="DeviceNet Interface Configuration", "DeviceNET in"=w335) -> ("error out"=w337:errorcluster, "DeviceNET out"=w342:refnum<class "DeviceNET.lvclass">)  [unwired: 7 in]
                      n135 = call-dynamic "Write Interface Name.vi"("error in (no error)"=w337, "Interface Name"="Interface Name", "DeviceNET in"=w342) -> ("error out"=w336:errorcluster, "DeviceNET out"=w341:refnum<class "DeviceNET.lvclass">)  [unwired: 7 in]
                      n136 = call-dynamic "Setup.vi"("protocol selection ref"=w333, "error in (no error)"=w336, "Comm master cluster in"=w334, "DeviceNET in"=w341) -> ("error out"=w344:errorcluster, "DeviceNET out"=w345:refnum<class "DeviceNET.lvclass">)  [unwired: 6 in]
                    }
                    frame Enabled {
                    }
                  }
                }
              }
            }
          }
        }
      }
      event Timeout {
        n137 = event-data() -> ()  [unwired: 1 in, 3 out]
      }
    }
  }
  "Read Completed" <- w8
